vi "FGV_SelectClass.vi"(7 "Action":enum16{"Set", "Get"}(ring)=enum."Get", 11 "EventMsg.lvclass":refnum<class "EventMsg.lvclass">) -> (3 "EventMsg.lvclass 2":refnum<class "EventMsg.lvclass">)   [LabVIEW 2014, in "EventMsg.lvclass"]
uses:
  EventMsg.lvclass
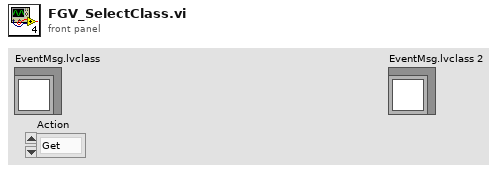
[diagram p1: front panel]
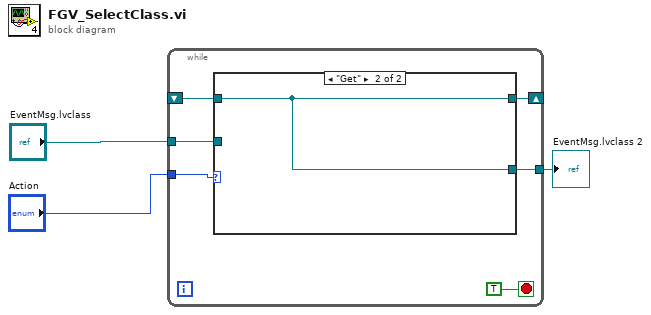
[diagram p0: block diagram]
diagram:
  n1 = while {
    tunnel: "EventMsg.lvclass" -> [w4]
    shift-right: [w5] -> _
    shift-left: _ -> [w6]
    tunnel: [w7] -> w2
    tunnel: "Action" -> [w8]
    stop <- TRUE stop-if-true
    n2 = case shown="\"Get\"" w8 {
      tunnel: [w10 w11] -> w7
      tunnel: w6 -> [_ w11]
      tunnel: [w10 w11] -> w5
      tunnel: w4 -> [w10 _]
      frame "Set", Default {
      }
      frame "Get" {
      }
    }
  }
  "EventMsg.lvclass 2" <- w2
